vi "Name.vi"() -> (2 "Name":string)   [LabVIEW 2020, in "_Template.lvlib" / "Templates.lvlib" / "TEMPLATE jettl Msg.lvlib" / "TEMPLATE.lvlib"]
uses:
  TEMPLATE.lvlib
  TEMPLATE Msg/TEMPLATE Msg/TEMPLATE Msg.lvclass
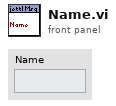
[diagram p1: front panel]
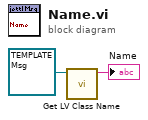
[diagram p0: block diagram]
diagram:
  n1 = call <vilib>:"Get LV Class Name.vi"("object"=refnum<class "TEMPLATE Msg.lvclass"> refnum ("_Template.lvlib:Templates.lvlib:TEMPLATE jettl Msg.lvlib:TEMPLATE Msg.lvlib:TEMPLATE Msg.lvclass")) -> ("class name"=→"Name":string)  [unwired: 9 in, 1 out]
